vi "Autonomous Independent.vi"() -> ()   [LabVIEW 2013]
doc: "This VI is called when autonomous begins, and will automatically be terminated when autonomous ends. You can carry out timed or sensor driven robot movement independently without needing to return to the caller."
uses:
  Robot Global Data.vi
  <vilib>/Rock Robotics/WPI/RobotDrive/WPI_RobotDriveGetSetRefNum.vi
  <vilib>/Rock Robotics/WPI/RobotDrive/WPI_RobotDriveArcadeDrive_Standard(NoSaturation).vi
  <vilib>/Rock Robotics/WPI/Joystick/WPI_JoystickGetSetRefNum.vi
panel:
  out "Current Movement, for debugging":T1 {"Y Joystick Value" scale=1.0..-1.0; "X Joystick Value" scale=-1.0..1.0}
  in  "Array of robot movements":T2(array[cluster]) {"Y Joystick Value" scale=1.0..-1.0; "X Joystick Value" scale=-1.0..1.0}
  # "Be sure to right-click and choose Data Operations>>Make Current Value default if you want to save the array values with the VI"
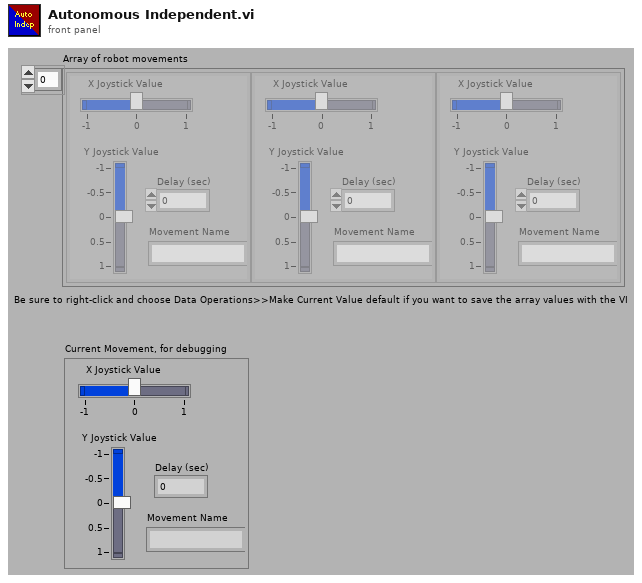
[diagram p1: front panel]
types:
  T1 = cluster{"X Joystick Value":dbl, "Y Joystick Value":dbl, "Delay (sec)":dbl, "Movement Name":string}
  T2 = cluster{"X Joystick Value":dbl, "Y Joystick Value":dbl, "Delay (sec)":dbl, "Movement Name":string}[]
  T3 = typedef "WPI_RobotDriveDevRef.ctl" = cluster{"DevStatus":errorcluster, "Motors[]":T4[], "Square Inputs":bool, "Max Output":dbl, "Isochronous":bool}
  T4 = typedef "WPI_MotorControlDeviceRef.ctl" = cluster{"DeviceStatus":errorcluster, "Type":enum16{"PWM", "CAN"}, "PWM":cluster{"Digital Module":T5, "PWM Channel":T6, "DeadBand":T7}, "CAN":cluster{"Device Number":u8, "Control Mode":T8, "Semaphore":T9, "Max Vout":dbl}, "Invert":bool, "TransformRef":T10, "InvTransformRef":T10}
  T5 = typedef "FPGA_TypedefDigitalModule.ctl" = enum16{"Digital Module 1", "Digital Module 2"}
  T6 = typedef "FPGA_DIOPWMChannel.ctl" = enum8{"PWM 1", "PWM 2", "PWM 3", "PWM 4", "PWM 5", "PWM 6", "PWM 7", "PWM 8", "PWM 9", "PWM 10", "Invalid"}
  T7 = typedef "WPI_PWMDeadband.ctl" = cluster{"Name":string, "maxPositivePwm":i32, "minPositivePwm":i32, "centerPwm":i32, "maxNegativePwm":i32, "minNegativePwm":i32, "angularRange":u16}
  T8 = typedef "WPI_CANJaguar_ControlMode.ctl" = enum8{"Percent VBus", "Current", "Speed", "Position", "Voltage"}
  T9 = typedef "Semaphore RefNum" = refnum<k1>
  T10 = typedef "WPI_PWMTransform_ConPane.ctl" = refnum<vi>
  T11 = typedef "WPI_JoystickDevRef.ctl" = cluster{"Device":T12}
  T12 = typedef "WPI_JoystickDeviceEnum.ctl" = enum16{"USB 1", "USB 2", "USB 3", "USB 4", "Kinect 1", "Kinect 2"}
  T13 = cluster{"axis 1 (x)":dbl, "axis 2 (y)":dbl, "axis 3 (throttle)":dbl, "axis 4":dbl, "axis 5":dbl, "axis 6":dbl}
  T14 = typedef "WPI_AnalogChannelDevRef.ctl" = cluster{"DevStatus":errorcluster, "Analog Module":T15, "Analog Channel":T16}
  T15 = typedef "FPGA_TypedefAnalogModule.ctl" = enum16{"Analog Module 1", "Analog Module 2"}
  T16 = typedef "FPGA_AIChannel.ctl" = enum8{"AI 1", "AI 2", "AI 3", "AI 4", "AI 5", "AI 6", "AI 7", "AI 8", "Invalid"}
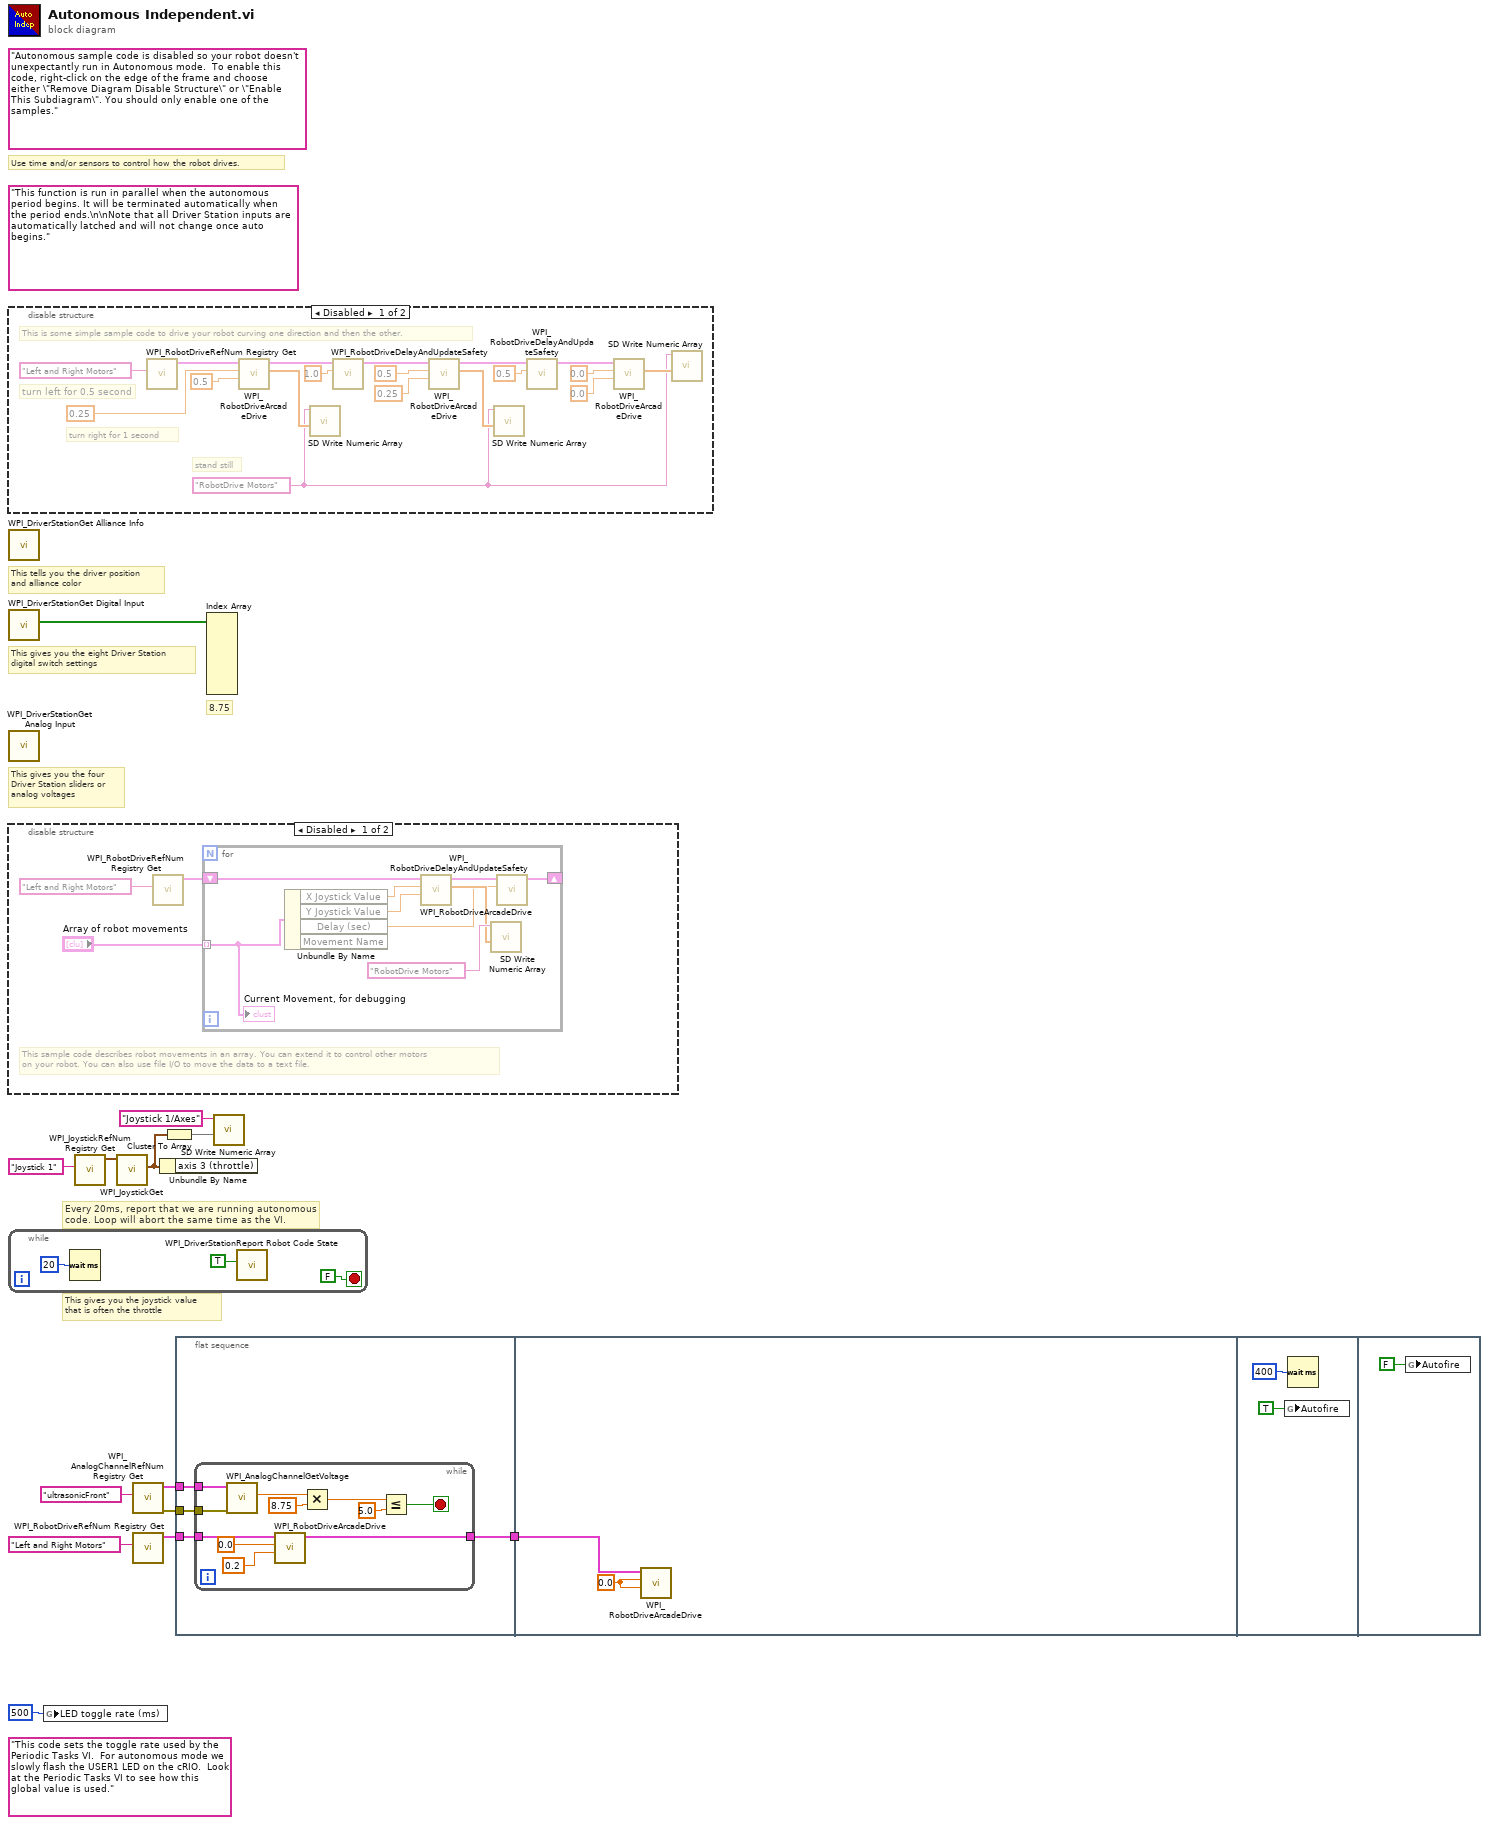
[diagram p0: block diagram]
diagram:
  (unwired) "This code sets the toggle rate used by the Periodic Tasks VI.  For autonomous mode we slowly flash the USER1 LED on the cRIO.  Look at the Periodic Tasks VI to see how this global value is used."
  (unwired) "Autonomous sample code is disabled so your robot doesn't unexpectantly run in Autonomous mode.  To enable this code, right-click on the edge of the frame and choose either \"Remove Diagram Disable Structure\" or \"Enable This Subdiagram\". You should only enable one of the samples."
  (unwired) "This function is run in parallel when the autonomous period begins. It will be terminated automatically when the period ends.\n\nNote that all Driver Station inputs are automatically latched and will not change once auto begins."
  # "8.75"
  # "Every 20ms, report that we are running autonomous\ncode. Loop will abort the same time as the VI."
  # "This gives you the joystick value\nthat is often the throttle"
  # "Use time and/or sensors to control how the robot drives."
  # "This tells you the driver position\nand alliance color"
  # "This gives you the eight Driver Station\ndigital switch settings"
  # "This gives you the four\nDriver Station sliders or\nanalog voltages"
  n1 = disable-structure shown="Disabled" {
    frame Disabled {
      w14 = "RobotDrive Motors" ("Name")
      # "This is some simple sample code to drive your robot curving one direction and then the other."
      # "stand still"
      # "turn left for 0.5 second"
      # "turn right for 1 second"
      n2 = call <vilib>:"WPI_RobotDriveRefNum Registry Get.vi"("refnum name"="Left and Right Motors") -> ("RobotDriveDevRef"=w18:T3)  [unwired: 1 in, 9 out]
      n3 = call-poly <vilib>:"WPI_RobotDriveArcadeDrive.vi"("Y axis value"=0.5 ("X axis value"), "X axis value"=0.25, "RobotDriveDevRef"=w18) -> ("Motor Values"=w17:dbl[], "RobotDriveDevRef"=w25:T3)  [unwired: 1 in, 6 out]
      n4 = call <vilib>:"SD Write Numeric Array.vi"("Numeric Array"=w17, "Name"=w14) -> ()  [unwired: 8 in, 2 out]
      n5 = call <vilib>:"WPI_RobotDriveDelayAndUpdateSafety.vi"("Delay (s)"=1.0, "RobotDriveDevRef"=w25) -> ("RobotDriveDevRef 2"=w24:T3)  [unwired: 8 in, 1 out]
      n6 = call-poly <vilib>:"WPI_RobotDriveArcadeDrive.vi"("Y axis value"=0.25 ("X axis value"), "X axis value"=0.5, "RobotDriveDevRef"=w24) -> ("Motor Values"=w16:dbl[], "RobotDriveDevRef"=w23:T3)  [unwired: 1 in, 6 out]
      n7 = call <vilib>:"SD Write Numeric Array.vi"("Numeric Array"=w16, "Name"=w14) -> ()  [unwired: 8 in, 2 out]
      n8 = call <vilib>:"WPI_RobotDriveDelayAndUpdateSafety.vi"("Delay (s)"=0.5, "RobotDriveDevRef"=w23) -> ("RobotDriveDevRef 2"=w22:T3)  [unwired: 8 in, 1 out]
      n9 = call-poly <vilib>:"WPI_RobotDriveArcadeDrive.vi"("Y axis value"=0.0 ("X axis value"), "X axis value"=0.0, "RobotDriveDevRef"=w22) -> ("Motor Values"=w15:dbl[])  [unwired: 1 in, 7 out]
      n10 = call <vilib>:"SD Write Numeric Array.vi"("Numeric Array"=w15, "Name"=w14) -> ()  [unwired: 8 in, 2 out]
    }
    frame Enabled {
    }
  }
  n11 = call <vilib>:"WPI_DriverStationGet Alliance Info.vi"() -> ()  [unwired: 12 out]
  n12 = call <vilib>:"WPI_DriverStationGet Digital Input.vi"() -> ("Driver Station Digital Input (1-8)"=w13:bool[])  [unwired: 11 out]
  n13 = call <vilib>:"WPI_DriverStationGet Analog Input.vi"() -> ()  [unwired: 12 out]
  n14 = disable-structure shown="Disabled" {
    frame Disabled {
      # "This sample code describes robot movements in an array. You can extend it to control other motors\non your robot. You can also use file I/O to move the data to a text file."
      n15 = call <vilib>:"WPI_RobotDriveRefNum Registry Get.vi"("refnum name"="Left and Right Motors") -> ("RobotDriveDevRef"=w33:T3)  [unwired: 1 in, 9 out]
      n16 = for {
        shift-right: [w39] -> _
        shift-left: w33 -> [w40]
        tunnel: "Array of robot movements" -> [w35] mode=indexing
        n17 = Unbundle By Name(w35) -> ("X Joystick Value"=w38:dbl, "Y Joystick Value"=w37:dbl, "Delay (sec)"=w36:dbl)  [unwired: 1 out]
        n18 = call-poly <vilib>:"WPI_RobotDriveArcadeDrive.vi"("Y axis value"=w37, "X axis value"=w38, "RobotDriveDevRef"=w40) -> ("Motor Values"=w42:dbl[], "RobotDriveDevRef"=w41:T3)  [unwired: 1 in, 6 out]
        n19 = call <vilib>:"SD Write Numeric Array.vi"("Numeric Array"=w42, "Name"="RobotDrive Motors") -> ()  [unwired: 8 in, 2 out]
        n20 = call <vilib>:"WPI_RobotDriveDelayAndUpdateSafety.vi"("Delay (s)"=w36, "RobotDriveDevRef"=w41) -> ("RobotDriveDevRef 2"=w39:T3)  [unwired: 8 in, 1 out]
        "Current Movement, for debugging" <- w35
      }
    }
    frame Enabled {
    }
  }
  n21 = while {
    stop <- FALSE stop-if-true
    n22 = Wait (ms)(milliseconds to wait=u32 20) -> ()  [unwired: 1 out]
    n23 = call <vilib>:"WPI_DriverStationReport Robot Code State.vi"("Autonomous"=TRUE) -> ()  [unwired: 10 in, 1 out]
  }
  n24 = global write "Robot Global Data.vi" "LED toggle rate (ms)"(u32 500 ("LED ms toggle rate")) -> ()
  n25 = call <vilib>:"WPI_JoystickRefNum Registry Get.vi"("refnum name"="Joystick 1") -> ("JoystickDevRef"=w11:T11)  [unwired: 1 in, 9 out]
  n26 = call <vilib>:"WPI_JoystickGet.vi"("JoystickDevRef"=w11) -> ("Axes"=w8:T13)  [unwired: 1 in, 5 out]
  n27 = call <vilib>:"WPI_AnalogChannelRefNum Registry Get.vi"("refnum name"="ultrasonicFront") -> ("error out"=w4:errorcluster, "AIDeviceRef"=w5:T14)  [unwired: 9 in]
  n28 = call <vilib>:"WPI_RobotDriveRefNum Registry Get.vi"("refnum name"="Left and Right Motors") -> ("RobotDriveDevRef"=w2:T3)  [unwired: 1 in, 9 out]
  n29 = Unbundle By Name(w8) -> ()  [unwired: 1 out]
  n30 = Cluster To Array(cluster=w8) -> (array=w9:dbl[])
  n31 = flat-sequence {
    tunnel: w5 -> [w50]
    tunnel: w4 -> [w49]
    tunnel: w2 -> [w48]
    tunnel: [w47] -> w1
    tunnel: w1 -> [w62]
    frame #0 {
      n32 = while {
        tunnel: w50 -> [w56]
        tunnel: w49 -> [w55]
        tunnel: w48 -> [w53]
        tunnel: [w51] -> w47
        stop <- w54 stop-if-true
        n33 = call <vilib>:"WPI_AnalogChannelGetVoltage.vi"("error in (no error)"=w55, "AIDeviceRef"=w56) -> ("Voltage"=w57:dbl)  [unwired: 7 in, 2 out]
        n34 = call-poly <vilib>:"WPI_RobotDriveArcadeDrive.vi"("Y axis value"=0.2 ("X axis value"), "X axis value"=0.0, "RobotDriveDevRef"=w53) -> ("RobotDriveDevRef"=w51:T3)  [unwired: 6 in, 2 out]
        n35 = Multiply(x=w57, y=8.75) -> (x*y=w59:dbl)
        n36 = Less Or Equal?(x=w59, y=5.0) -> (x <= y?=w54:bool)
      }
    }
    frame #1 {
      w63 = 0.0 ("X axis value")
      n37 = call-poly <vilib>:"WPI_RobotDriveArcadeDrive.vi"("Y axis value"=w63, "X axis value"=w63, "RobotDriveDevRef"=w62) -> ()  [unwired: 6 in, 3 out]
    }
    frame #2 {
      n38 = global write "Robot Global Data.vi" "Autofire"(TRUE ("Autofire")) -> ()
      n39 = Wait (ms)(milliseconds to wait=u32 400) -> ()  [unwired: 1 out]
    }
    frame #3 {
      n40 = global write "Robot Global Data.vi" "Autofire"(FALSE ("Autofire")) -> ()
    }
  }
  n41 = Index Array(array=w13) -> ()  [unwired: 8 in, 8 out]
  n42 = call <vilib>:"SD Write Numeric Array.vi"("Numeric Array"=w9, "Name"="Joystick 1/Axes") -> ()  [unwired: 8 in, 2 out]
